vi "ADXL335.vi"() -> ()   [LabVIEW 2019]
uses:
  <vilib>/MakerHub/LINX/LMH-LINX.lvlib
  <vilib>/MakerHub/LINX/Public/Peripherals/Analog/Analog Read N Chans.vi
  <vilib>/MakerHub/LINX/Public/Utilities/Open Serial.vi
panel:
  out "Meter 3":dbl(knob) scale=0.0..5.0
  out "Meter 2":dbl(knob) scale=0.0..5.0
  out "Meter":dbl(knob) scale=0.0..5.0
  in  "stop":bool
  in  "Serial Port":refnum<visa-resource-name>="N/A"
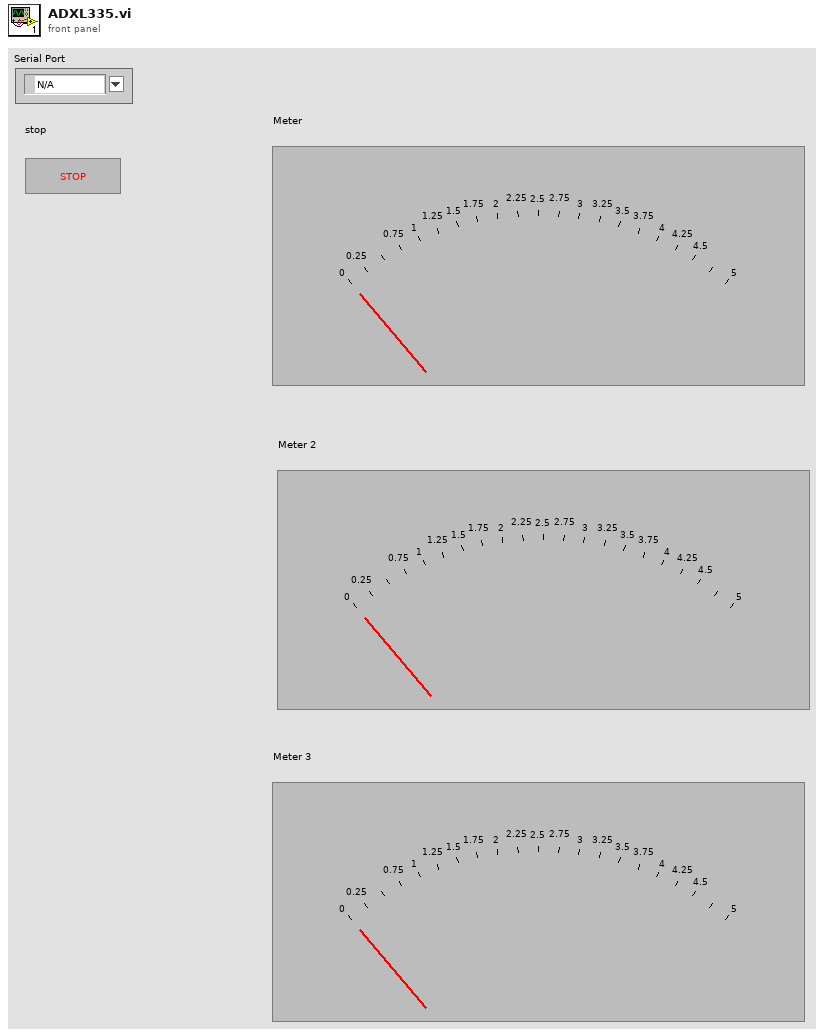
[diagram p1: front panel]
types:
  T1 = typedef "LMH-LINX.lvlib/LINX Ref.ctl" = cluster{"IO":T2, "Interface":T3, "LINX Device Config":T4}
  T2 = typedef "LMH-LINX.lvlib/Platform.ctl" = enum16{"Remote", "Local"}
  T3 = typedef "LMH-LINX.lvlib/Interface.ctl" = enum16{"Serial", "TCP"}
  T4 = typedef "LMH-LINX.lvlib/Device.lvlib/LINX Device Config.ctl" = cluster{"Interface":T3, "COM Port":refnum<visa-resource-name>, "TCP Configuration":T5, "Device Family":u8, "Device ID":u8, "Device Name":string, "TCP Ref":refnum<k5>, "Channels":T6}
  T5 = typedef "LMH-LINX.lvlib/Device.lvlib/TCP Config.ctl" = cluster{"IP Address":string, "Port":u16}
  T6 = typedef "LMH-LINX.lvlib/Channels.ctl" = cluster{"DI":u8[], "DO":u8[], "AI":u8[], "AO":u8[], "PWM":u8[], "QE":u8[], "UART":u8[], "I2C 2":u8[], "SPI":u8[], "CAN":u8[], "Servo":u8[], "AI Ref (V)":dbl, "AI Resolution (Bits)":u8, "AO Ref (V)":dbl, "AO Resolution (Bits)":u8}
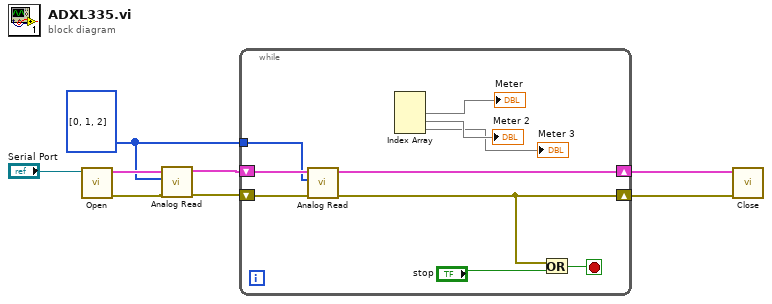
[diagram p0: block diagram]
diagram:
  w1 = u8[] [0, 1, 2] ("AI Channel(s)")
  n1 = call-poly <vilib>:"Open.vi"("Serial Port"="Serial Port") -> ("Error Out"=w3:errorcluster, "LINX Resource"=w5:T1)  [unwired: 8 in, 1 out]
  n2 = call-poly <vilib>:"Analog Read.vi"("Error In"=w3, "AI Channel(s)"=w1, "LINX Resource"=w5) -> ("Error Out"=w2:errorcluster, "LINX Resource"=w4:T1)  [unwired: 5 in, 2 out]
  n3 = while {
    shift-right: [w16] -> w7
    shift-left: w4 -> [w18]
    shift-right: [w15] -> w6
    shift-left: w2 -> [w17]
    tunnel: w1 -> [w12]
    stop <- w13 stop-if-true
    n4 = call-poly <vilib>:"Analog Read.vi"("Error In"=w17, "AI Channel(s)"=w12, "LINX Resource"=w18) -> ("Error Out"=w15:errorcluster, "LINX Resource"=w16:T1)  [unwired: 5 in, 2 out]
    n5 = Index Array() -> (element #1=→"Meter", element #2=→"Meter 2", element #3=→"Meter 3")  [unwired: 4 in]
    n6 = Or(x=w15, y="stop") -> (x .or. y?=w13:bool)
  }
  n7 = call <vilib>:"Close.vi"("Error In"=w6, "LINX Resource"=w7) -> ()  [unwired: 9 in, 1 out]
